vi "encoder_FPGA.vi"() -> ()   [LabVIEW 2019]
uses:
  <vilib>/rvi/Emulation/niFpgaGetClockAttributes.vi
  <vilib>/rvi/Emulation/niFpgaSctlEmulationGetInTimedLoop.vi
  <vilib>/rvi/Emulation/niFpgaEmulationReportErrorSimple.vi
  <vilib>/rvi/Emulation/niFpgaProcessEmulError.vi
  <vilib>/rvi/eio/common/nirviEmuTemplateMethod_errors.vi
  <vilib>/rvi/Emulation/niFpgaCriticalErrorInLSC.vi
  <vilib>/eio/EIONode/EIONode.xnode
panel:
  out "camera":bool
  in  "R_dir":bool
  in  "L_dir":bool
  in  "R_pwm input":i32
  in  "R_encoder reset":bool
  out "R_Encoder  (4x)":i32
  in  "tir_pwm input(escon)":i32
  in  "tir_DIR":bool
  in  "tir_Enable (escon)":bool
  in  "tir_stop":bool
  in  "tir_encoder reset":bool
  out "tir_Encoder  (4x)":i32
  in  "angle_pwm input(escon)":i32
  in  "angle_DIR":bool
  in  "angle_Enable (escon)":bool
  in  "angle_stop":bool
  in  "angle_encoder reset":bool
  out "angle_Encoder  (4x)":i32
  in  "직동_dir":bool
  in  "직동_pwm input":i32
  in  "pwm input":i32
  out "Encoder  (4x)":i32
  in  "encoder reset":bool
  in  "stop":bool
  # "오른쪽 바퀴 모터"
  # "왼쪽 바퀴 모터"
  # "직동 모터"
  # "trigger 모터"
  # "angle 모터"
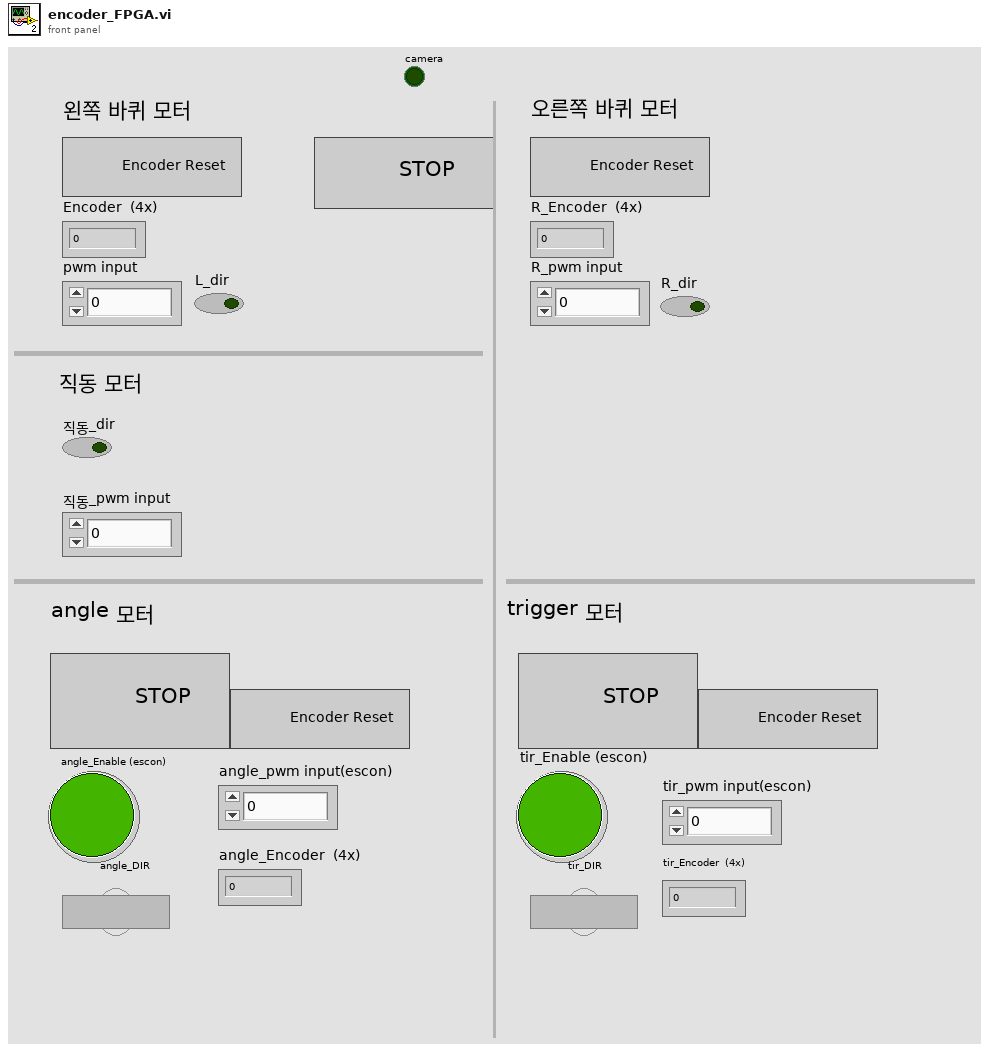
[diagram p1: front panel]
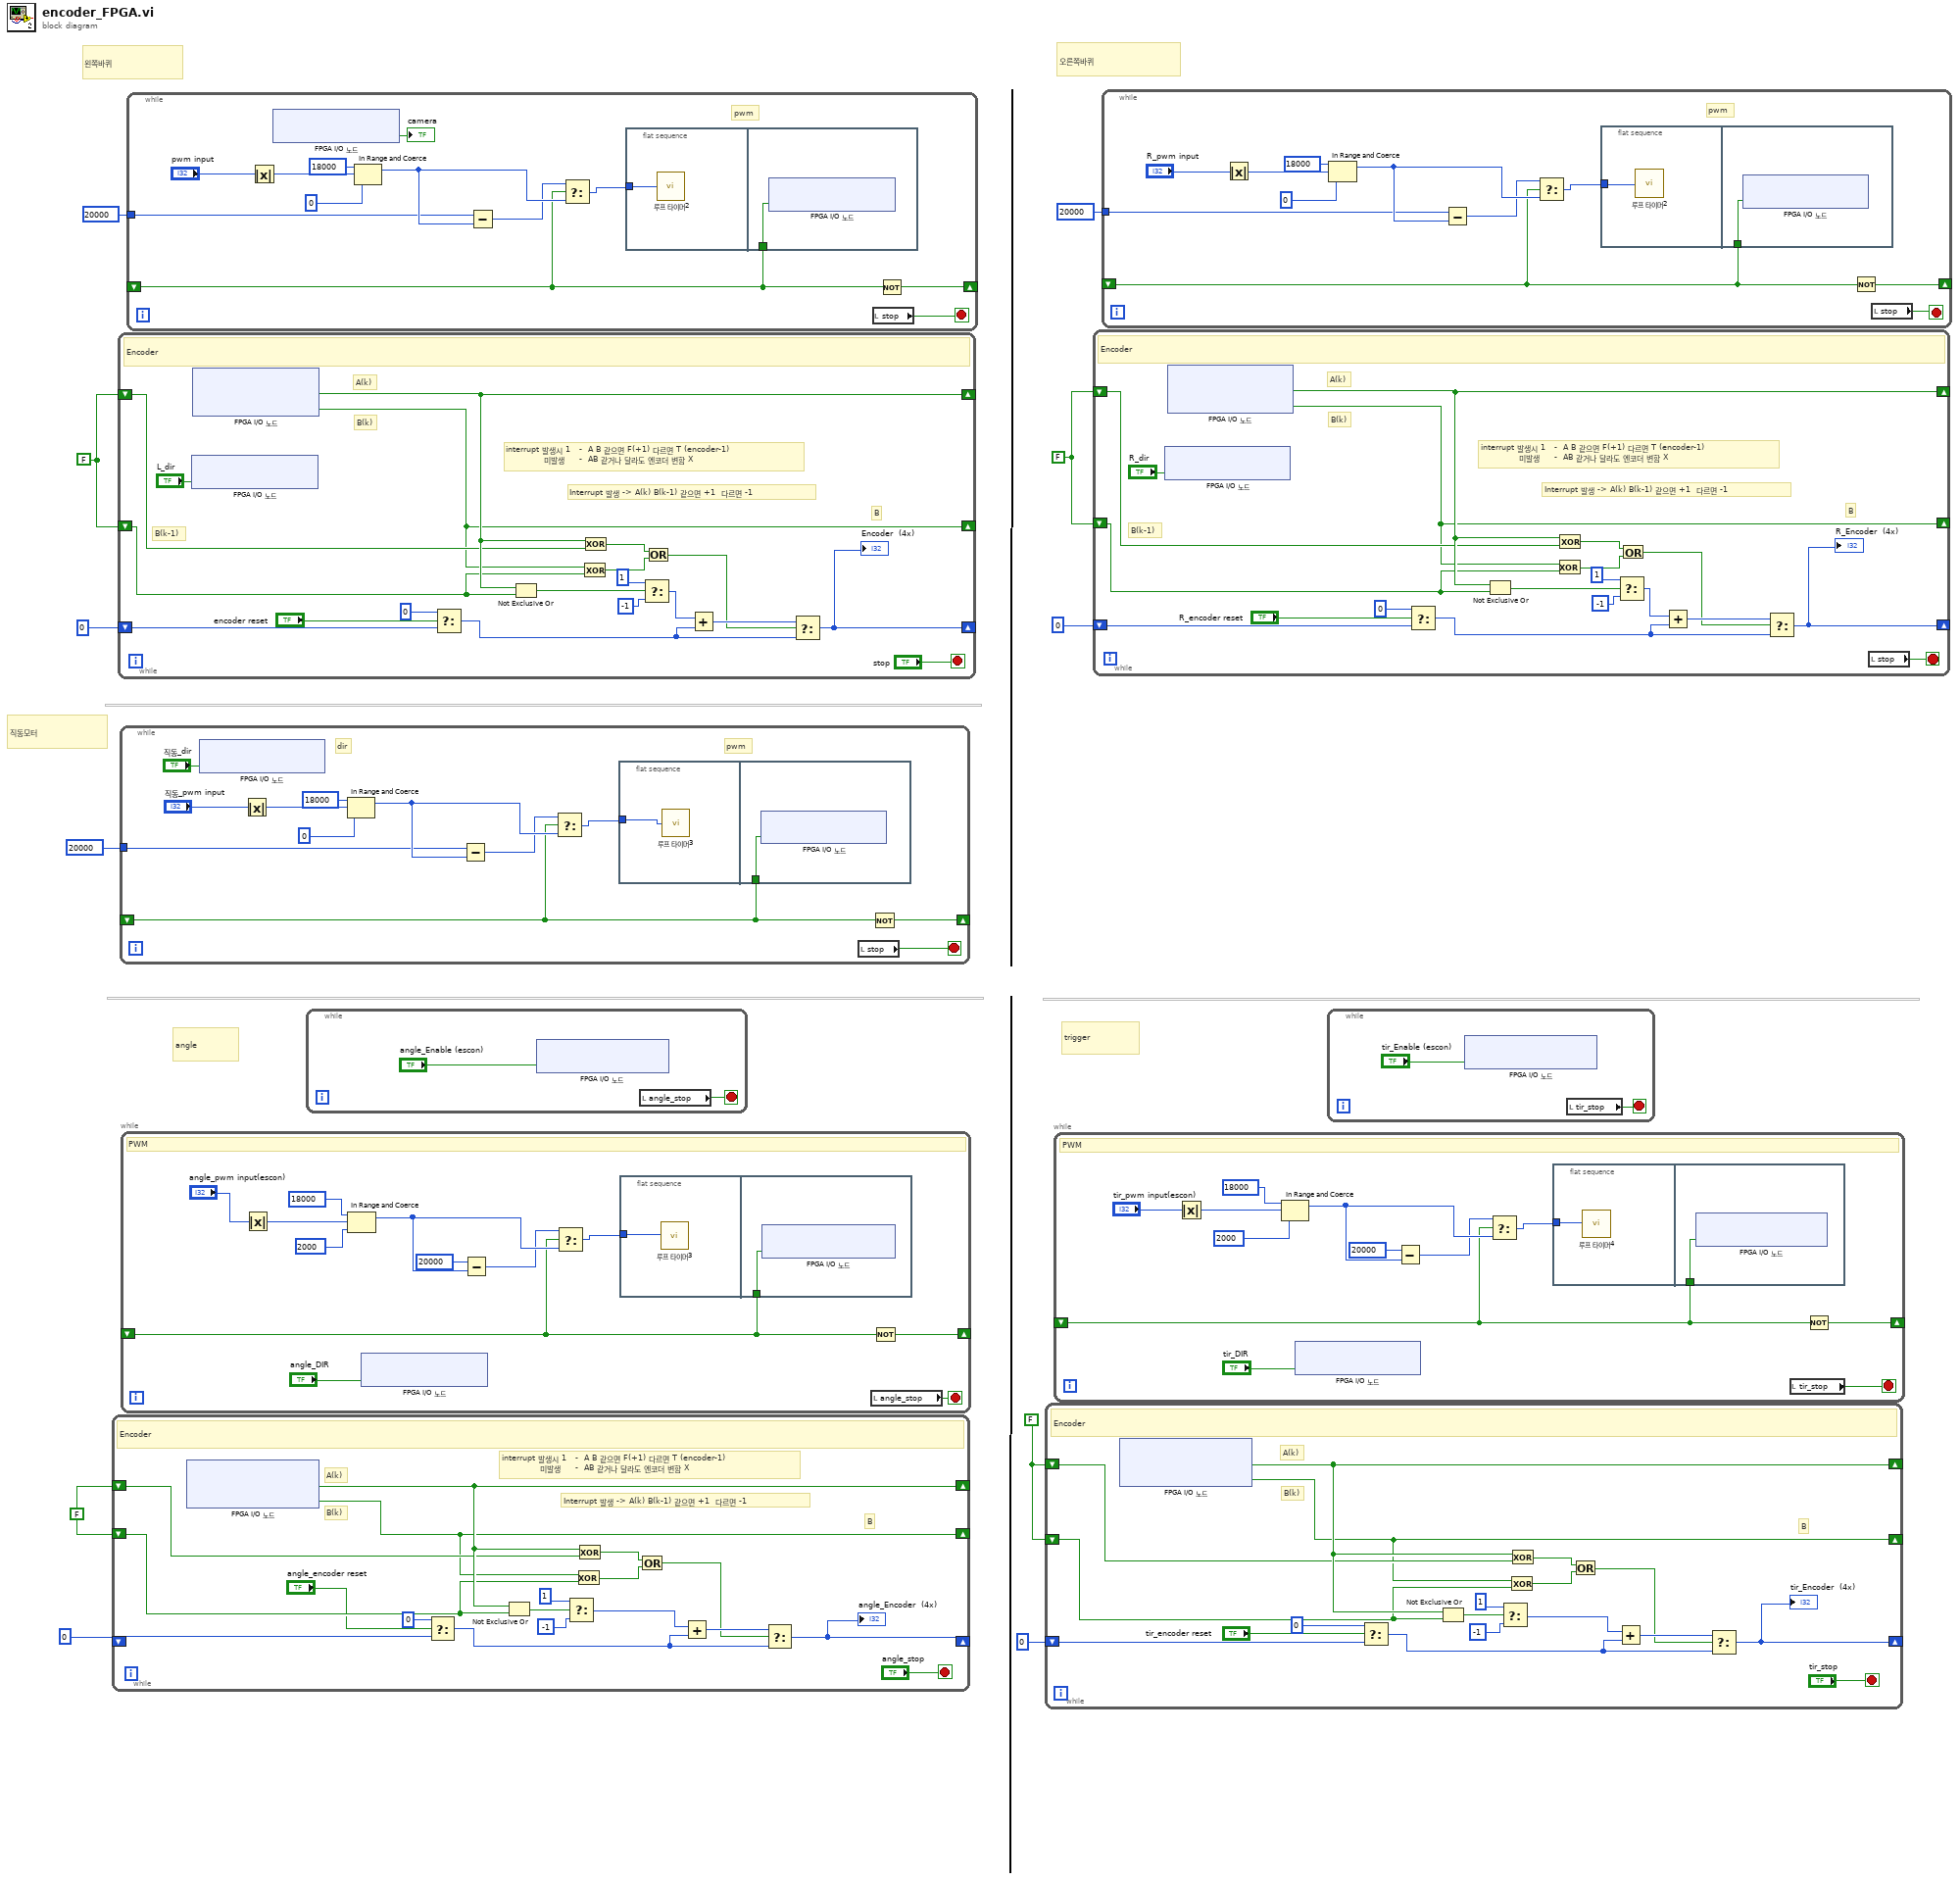
[diagram p0: block diagram]
diagram:
  w2 = FALSE
  w5 = FALSE
  w7 = FALSE
  w10 = FALSE
  # "오른쪽바퀴"
  # "왼쪽바퀴"
  # "trigger"
  # "angle"
  # "직동모터"
  n1 = while {
    shift-right: [w21] -> _
    shift-left: w7 -> [w20]
    shift-right: [w19] -> _
    shift-left: w7 -> [w18]
    shift-right: [w13] -> _
    shift-left: 0 -> [w12]
    stop <- "angle_stop" stop-if-true
    # "B"
    # "Interrupt 발생 -> A(k) B(k-1) 같으면 +1  다르면 -1"
    # "B(k)"
    # "A(k)"
    # "interrupt 발생시 1   -  A B 같으면 F(+1) 다르면 T (encoder-1)\n             미발생     -  AB 같거나 달라도 엔코더 변함 X"
    # "Encoder"
    n2 = xnode "FPGA I/O 노드"() -> ("ConnectorA/DIO9"=w21:bool, "ConnectorA/DIO10"=w19:bool)  [unwired: 2 in, 2 out]
    n3 = Select(t=0, s="angle_encoder reset", f=w12) -> (s? t:f=w16:i32)
    n4 = Not Exclusive Or(1:w18, 2:w21) -> (0:w27:bool)
    n5 = Select(t=i16 1, s=w27, f=i16 -1) -> (s? t:f=w26:i16)
    n6 = Exclusive Or(1:w18, 2:w19) -> (0:w23:bool)
    n7 = Exclusive Or(1:w20, 2:w21) -> (0:w24:bool)
    n8 = Or(x=w24, y=w23) -> (x .or. y?=w22:bool)
    n9 = Add(x=w26, y=w16) -> (x+y=w25:i32)
    n10 = Select(t=w25, s=w22, f=w16) -> (s? t:f=w13:i32)
    "angle_Encoder  (4x)" <- w13
  }
  n11 = while {
    shift-right: [w40] -> _
    shift-left: w10 -> [w39]
    shift-right: [w38] -> _
    shift-left: w10 -> [w37]
    shift-right: [w32] -> _
    shift-left: 0 -> [w31]
    stop <- "stop" stop-if-true
    # "B"
    # "B(k-1)"
    # "Interrupt 발생 -> A(k) B(k-1) 같으면 +1  다르면 -1"
    # "B(k)"
    # "A(k)"
    # "interrupt 발생시 1   -  A B 같으면 F(+1) 다르면 T (encoder-1)\n             미발생     -  AB 같거나 달라도 엔코더 변함 X"
    # "Encoder"
    n12 = xnode "FPGA I/O 노드"("ConnectorA/DIO3"="L_dir") -> ()  [unwired: 1 in, 1 out]
    n13 = xnode "FPGA I/O 노드"() -> ("ConnectorA/DIO0"=w40:bool, "ConnectorA/DIO1"=w38:bool)  [unwired: 2 in, 2 out]
    n14 = Select(t=0, s="encoder reset", f=w31) -> (s? t:f=w35:i32)
    n15 = Not Exclusive Or(1:w37, 2:w40) -> (0:w46:bool)
    n16 = Exclusive Or(1:w37, 2:w38) -> (0:w42:bool)
    n17 = Exclusive Or(1:w39, 2:w40) -> (0:w43:bool)
    n18 = Select(t=i16 1, s=w46, f=i16 -1) -> (s? t:f=w45:i16)
    n19 = Or(x=w43, y=w42) -> (x .or. y?=w41:bool)
    n20 = Add(x=w45, y=w35) -> (x+y=w44:i32)
    n21 = Select(t=w44, s=w41, f=w35) -> (s? t:f=w32:i32)
    "Encoder  (4x)" <- w32
  }
  n22 = while {
    shift-right: [w55] -> _
    shift-left: _ -> [w54]
    tunnel: 20000 ("T(escon)") -> [w53]
    stop <- w50 stop-if-true
    # "dir"
    # "pwm"
    n23 = xnode "FPGA I/O 노드"("ConnectorB/DIO6"="직동_dir") -> ()  [unwired: 1 in, 1 out]
    n24 = Absolute Value(x="직동_pwm input") -> (abs(x)=w60:i32)
    n25 = In Range and Coerce(upper limit=i16 18000, x=w60, lower limit=i16 0) -> (coerced(x)=w58:i32)  [unwired: 1 out]
    n26 = Subtract(x=w53, y=w58) -> (x-y=w57:i32)
    n27 = Select(t=w57, s=w54, f=w58) -> (s? t:f=w56:i32)
    n28 = flat-sequence {
      tunnel: w56 -> [w61]
      tunnel: w54 -> [w62]
      frame #0 {
        n29 = call "루프 타이머3"("Count(Ticks)"=w61) -> ()  [unwired: 1 out]
      }
      frame #1 {
        n30 = xnode "FPGA I/O 노드"("ConnectorB/DIO5"=w62) -> ()  [unwired: 1 in, 1 out]
      }
    }
    n31 = local read "stop"() -> (w50:bool)
    n32 = Not(x=w54) -> (.not. x?=w55:bool)
  }
  n33 = while {
    shift-right: [w69] -> _
    shift-left: _ -> [w68]
    stop <- w65 stop-if-true
    # "PWM"
    n34 = Absolute Value(x="angle_pwm input(escon)") -> (abs(x)=w74:i32)
    n35 = In Range and Coerce(upper limit=i16 18000, x=w74, lower limit=i16 2000) -> (coerced(x)=w72:i32)  [unwired: 1 out]
    n36 = xnode "FPGA I/O 노드"("ConnectorA/DIO8"="angle_DIR") -> ()  [unwired: 1 in, 1 out]
    n37 = Subtract(x=20000, y=w72) -> (x-y=w71:i32)
    n38 = Select(t=w71, s=w68, f=w72) -> (s? t:f=w70:i32)
    n39 = flat-sequence {
      tunnel: w70 -> [w75]
      tunnel: w68 -> [w76]
      frame #0 {
        n40 = call "루프 타이머3"("Count(Ticks)"=w75) -> ()  [unwired: 1 out]
      }
      frame #1 {
        n41 = xnode "FPGA I/O 노드"("ConnectorA/DIO14"=w76) -> ()  [unwired: 1 in, 1 out]
      }
    }
    n42 = local read "angle_stop"() -> (w65:bool)
    n43 = Not(x=w68) -> (.not. x?=w69:bool)
  }
  n44 = while {
    shift-right: [w83] -> _
    shift-left: _ -> [w82]
    tunnel: 20000 ("T(escon)") -> [w81]
    stop <- w78 stop-if-true
    # "pwm"
    n45 = Absolute Value(x="pwm input") -> (abs(x)=w88:i32)
    n46 = xnode "FPGA I/O 노드"() -> ("ConnectorA/DIO4"=→"camera":bool)  [unwired: 1 in, 1 out]
    n47 = In Range and Coerce(upper limit=i16 18000, x=w88, lower limit=i16 0) -> (coerced(x)=w86:i32)  [unwired: 1 out]
    n48 = Subtract(x=w81, y=w86) -> (x-y=w85:i32)
    n49 = Select(t=w85, s=w82, f=w86) -> (s? t:f=w84:i32)
    n50 = flat-sequence {
      tunnel: w84 -> [w89]
      tunnel: w82 -> [w90]
      frame #0 {
        n51 = call "루프 타이머2"("Count(Ticks)"=w89) -> ()  [unwired: 1 out]
      }
      frame #1 {
        n52 = xnode "FPGA I/O 노드"("ConnectorA/DIO2"=w90) -> ()  [unwired: 1 in, 1 out]
      }
    }
    n53 = local read "stop"() -> (w78:bool)
    n54 = Not(x=w82) -> (.not. x?=w83:bool)
  }
  n55 = while {
    stop <- w91 stop-if-true
    n56 = xnode "FPGA I/O 노드"("ConnectorA/DIO15"="angle_Enable (escon)") -> ()  [unwired: 1 in, 1 out]
    n57 = local read "angle_stop"() -> (w91:bool)
  }
  n58 = while {
    shift-right: [w102] -> _
    shift-left: w5 -> [w101]
    shift-right: [w100] -> _
    shift-left: w5 -> [w99]
    shift-right: [w94] -> _
    shift-left: 0 -> [w93]
    stop <- "tir_stop" stop-if-true
    # "B"
    # "B(k)"
    # "A(k)"
    # "Encoder"
    n59 = xnode "FPGA I/O 노드"() -> ("ConnectorB/DIO9"=w102:bool, "ConnectorB/DIO10"=w100:bool)  [unwired: 2 in, 2 out]
    n60 = Select(t=0, s="tir_encoder reset", f=w93) -> (s? t:f=w97:i32)
    n61 = Not Exclusive Or(1:w99, 2:w102) -> (0:w108:bool)
    n62 = Select(t=i16 1, s=w108, f=i16 -1) -> (s? t:f=w107:i16)
    n63 = Exclusive Or(1:w99, 2:w100) -> (0:w104:bool)
    n64 = Exclusive Or(1:w101, 2:w102) -> (0:w105:bool)
    n65 = Or(x=w105, y=w104) -> (x .or. y?=w103:bool)
    n66 = Add(x=w107, y=w97) -> (x+y=w106:i32)
    n67 = Select(t=w106, s=w103, f=w97) -> (s? t:f=w94:i32)
    "tir_Encoder  (4x)" <- w94
  }
  n68 = while {
    shift-right: [w117] -> _
    shift-left: _ -> [w116]
    stop <- w113 stop-if-true
    # "PWM"
    n69 = Absolute Value(x="tir_pwm input(escon)") -> (abs(x)=w122:i32)
    n70 = In Range and Coerce(upper limit=i16 18000, x=w122, lower limit=i16 2000) -> (coerced(x)=w120:i32)  [unwired: 1 out]
    n71 = xnode "FPGA I/O 노드"("ConnectorB/DIO8"="tir_DIR") -> ()  [unwired: 1 in, 1 out]
    n72 = Subtract(x=20000, y=w120) -> (x-y=w119:i32)
    n73 = Select(t=w119, s=w116, f=w120) -> (s? t:f=w118:i32)
    n74 = flat-sequence {
      tunnel: w118 -> [w123]
      tunnel: w116 -> [w124]
      frame #0 {
        n75 = call "루프 타이머4"("Count(Ticks)"=w123) -> ()  [unwired: 1 out]
      }
      frame #1 {
        n76 = xnode "FPGA I/O 노드"("ConnectorB/DIO14"=w124) -> ()  [unwired: 1 in, 1 out]
      }
    }
    n77 = local read "tir_stop"() -> (w113:bool)
    n78 = Not(x=w116) -> (.not. x?=w117:bool)
  }
  n79 = while {
    shift-right: [w135] -> _
    shift-left: w2 -> [w134]
    shift-right: [w133] -> _
    shift-left: w2 -> [w132]
    shift-right: [w128] -> _
    shift-left: 0 -> [w127]
    stop <- w126 stop-if-true
    # "B"
    # "B(k-1)"
    # "Interrupt 발생 -> A(k) B(k-1) 같으면 +1  다르면 -1"
    # "B(k)"
    # "A(k)"
    # "interrupt 발생시 1   -  A B 같으면 F(+1) 다르면 T (encoder-1)\n             미발생     -  AB 같거나 달라도 엔코더 변함 X"
    # "Encoder"
    n80 = xnode "FPGA I/O 노드"("ConnectorB/DIO3"="R_dir") -> ()  [unwired: 1 in, 1 out]
    n81 = xnode "FPGA I/O 노드"() -> ("ConnectorB/DIO0"=w135:bool, "ConnectorB/DIO1"=w133:bool)  [unwired: 2 in, 2 out]
    n82 = Select(t=0, s="R_encoder reset", f=w127) -> (s? t:f=w131:i32)
    n83 = Not Exclusive Or(1:w132, 2:w135) -> (0:w141:bool)
    n84 = Exclusive Or(1:w132, 2:w133) -> (0:w137:bool)
    n85 = Exclusive Or(1:w134, 2:w135) -> (0:w138:bool)
    n86 = Select(t=i16 1, s=w141, f=i16 -1) -> (s? t:f=w140:i16)
    n87 = Or(x=w138, y=w137) -> (x .or. y?=w136:bool)
    n88 = Add(x=w140, y=w131) -> (x+y=w139:i32)
    n89 = Select(t=w139, s=w136, f=w131) -> (s? t:f=w128:i32)
    "R_Encoder  (4x)" <- w128
    n90 = local read "stop"() -> (w126:bool)
  }
  n91 = while {
    shift-right: [w149] -> _
    shift-left: _ -> [w148]
    tunnel: 20000 ("T(escon)") -> [w147]
    stop <- w144 stop-if-true
    # "pwm"
    n92 = Absolute Value(x="R_pwm input") -> (abs(x)=w154:i32)
    n93 = In Range and Coerce(upper limit=i16 18000, x=w154, lower limit=i16 0) -> (coerced(x)=w152:i32)  [unwired: 1 out]
    n94 = Subtract(x=w147, y=w152) -> (x-y=w151:i32)
    n95 = Select(t=w151, s=w148, f=w152) -> (s? t:f=w150:i32)
    n96 = flat-sequence {
      tunnel: w150 -> [w155]
      tunnel: w148 -> [w156]
      frame #0 {
        n97 = call "루프 타이머2"("Count(Ticks)"=w155) -> ()  [unwired: 1 out]
      }
      frame #1 {
        n98 = xnode "FPGA I/O 노드"("ConnectorB/DIO2"=w156) -> ()  [unwired: 1 in, 1 out]
      }
    }
    n99 = Not(x=w148) -> (.not. x?=w149:bool)
    n100 = local read "stop"() -> (w144:bool)
  }
  n101 = while {
    stop <- w157 stop-if-true
    n102 = xnode "FPGA I/O 노드"("ConnectorB/DIO15"="tir_Enable (escon)") -> ()  [unwired: 1 in, 1 out]
    n103 = local read "tir_stop"() -> (w157:bool)
  }
